vi "PH_PLH-AccessInformation.set information.vi"(1 "error in(no error)":errorcluster, 2 "Mode":T1(ring)) -> (0 "error out":errorcluster)   [LabVIEW 2014, in "PH_PLH-AccessInformation.lvlib"]
doc: "This VI writes the infoation to the O-drive."
uses:
  PH_PLH-AccessInformation.lvlib
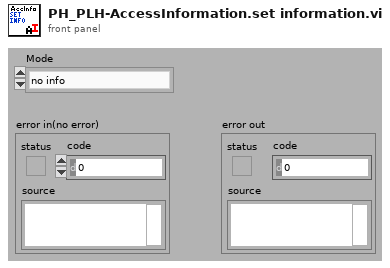
[diagram p1: front panel]
types:
  T1 = enum16{"no info", "free access", "Searchmode", "Shotmode"}
  T2 = enum16{"open", "replace", "create", "open or create", "replace or create", "replace or create with confirmation"}
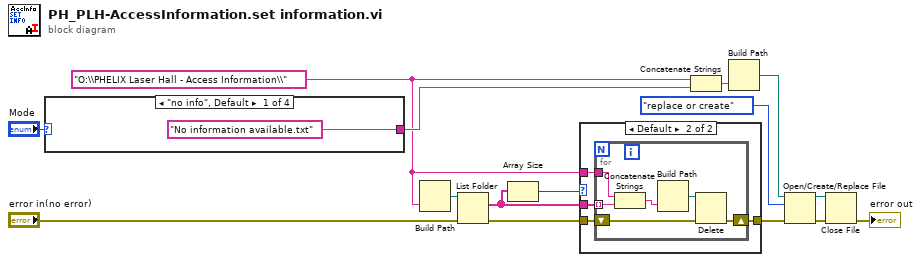
[diagram p0: block diagram]
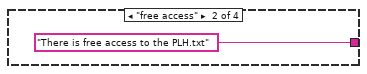
[diagram p3: hidden frame]
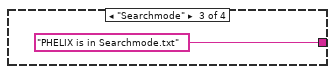
[diagram p4: hidden frame]
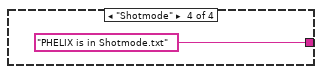
[diagram p5: hidden frame]
diagram:
  w9 = "O:\\PHELIX Laser Hall - Access Information\\" ("Path 2")
  n1 = case shown="\"no info\", Default" "Mode" {
    tunnel: ["No information available.txt" ("string") "There is free access to the PLH.txt" ("string") "PHELIX is in Searchmode.txt" ("string") "PHELIX is in Shotmode.txt" ("string")] -> w13
    frame "no info", Default {
    }
    frame "free access" {
    }
    frame "Searchmode" {
    }
    frame "Shotmode" {
    }
  }
  n2 = Build Path(name or relative path=w9) -> (appended path=w12:path)  [unwired: 1 in]
  n3 = List Folder(path=w12, error in="error in(no error)") -> (filenames=w11:string[], error out=w8:errorcluster)  [unwired: 2 in, 2 out]
  n4 = Array Size(array=w11) -> (size(s)=w10:i32)
  n5 = case shown="Default" w10 {
    tunnel: w8 -> [w20 w24]
    tunnel: [w20 w23] -> w2
    tunnel: w11 -> [_ w22]
    tunnel: w9 -> [_ w21]
    frame 0 {
    }
    frame Default {
      n6 = for {
        shift-right: [w29] -> w23
        shift-left: w24 -> [w30]
        tunnel: w22 -> [w26] mode=indexing
        tunnel: w21 -> [w27]
        n7 = Concatenate Strings(w27, w26) -> (w25:string)
        n8 = Build Path(name or relative path=w25) -> (appended path=w28:path)  [unwired: 1 in]
        n9 = Delete(path (use dialog)=w28, error in=w30) -> (error out=w29:errorcluster)  [unwired: 3 in, 2 out]
      }
    }
  }
  n10 = Concatenate Strings(w9, w13) -> (w3:string)
  n11 = Build Path(name or relative path=w3) -> (appended path=w6:path)  [unwired: 1 in]
  n12 = Open/Create/Replace File(file path (use dialog)=w6, error in=w2, operation (0:open)=T2."replace or create") -> (refnum out=w4:refnum<file>, error out=w5:errorcluster)  [unwired: 3 in, 1 out]
  n13 = Close File(refnum=w4, error in=w5) -> (error out=→"error out":errorcluster)  [unwired: 1 out]
